vi "手动调试界面.vi"() -> ()   [LabVIEW 2016, in "质控单元.lvlib"]
uses:
  <vilib>/Utility/miscctls.llb/LVPointTypeDef.ctl
panel:
  in  "加标回收流程":bool
  in  "关闭":bool
  in  "总氮停止":bool
  in  "总氮排液":bool
  in  "总氮调试":bool
  in  "CODCr停止":bool
  in  "CODCr排液":bool
  in  "CODCr调试":bool
  in  "CODMn停止":bool
  in  "CODMn排液":bool
  in  "CODMn调试":bool
  in  "总磷停止":bool
  in  "总磷排液":bool
  in  "总磷调试":bool
  in  "氨氮停止":bool
  in  "氨氮排液":bool
  in  "氨氮调试":bool
  # "手动调试界面"
  # "氨氮模块"
  # "总磷模块"
  # "总氮模块"
  # "CODMn模块"
  # "CODCr模块"
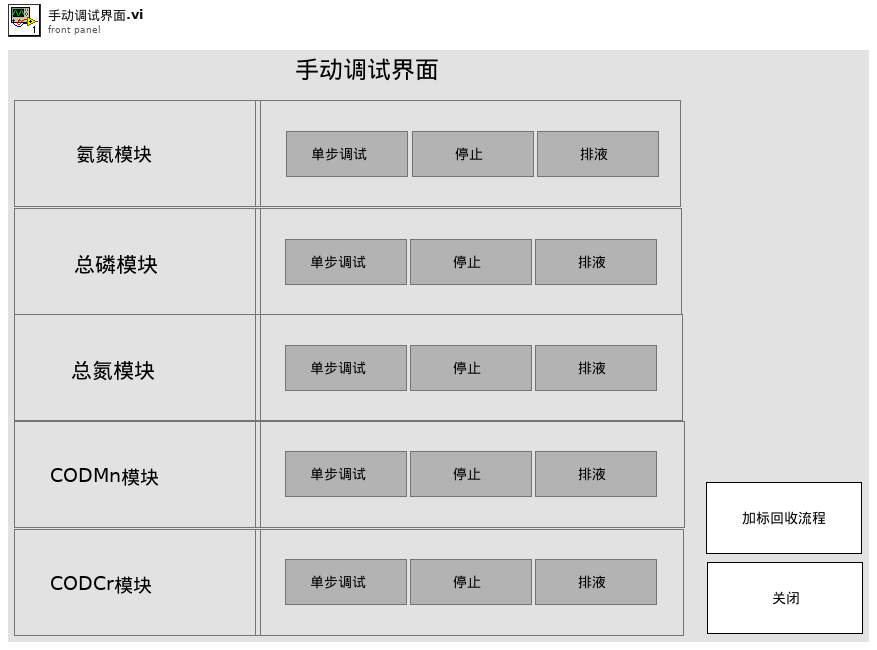
[diagram p1: front panel]
types:
  T1 = typedef "LVPointTypeDef.ctl" = cluster{"Horizontal":i16, "Vertical":i16}
  T2 = cluster{"氨氮":bool, "总磷":bool, "总氮":bool, "CODMn":bool, "CODCr":bool}
  T3 = enum32{"Bad", "Idle", "Run top level", "Running"}
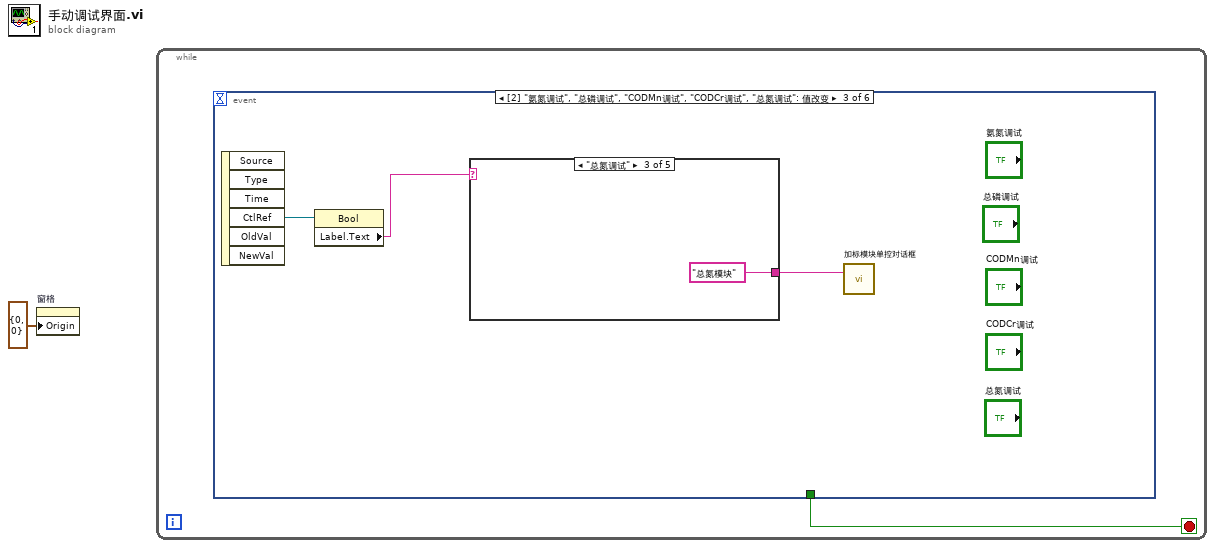
[diagram p0: block diagram]
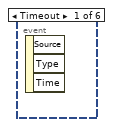
[diagram p2: hidden frame]
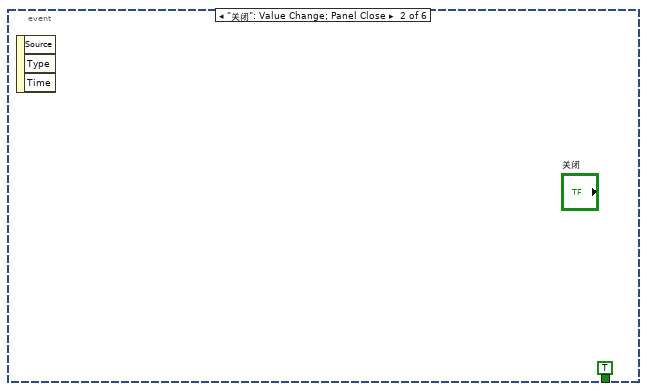
[diagram p3: hidden frame]
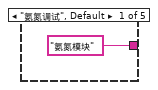
[diagram p4: hidden frame]
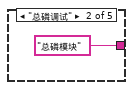
[diagram p5: hidden frame]
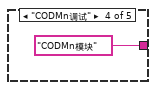
[diagram p6: hidden frame]
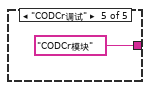
[diagram p7: hidden frame]
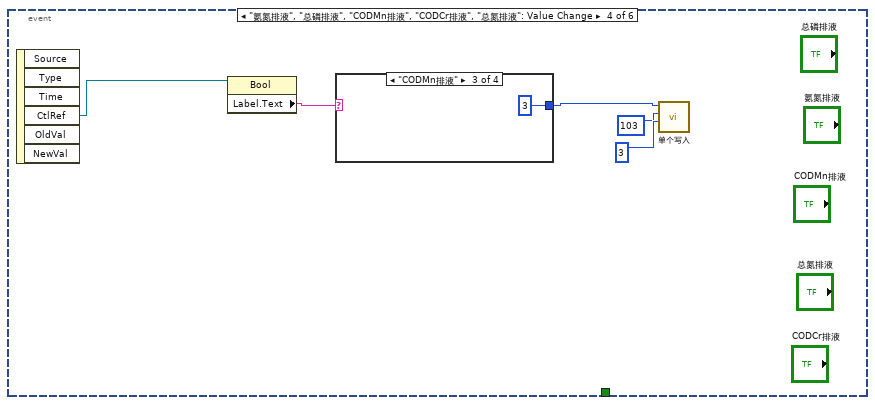
[diagram p8: hidden frame]
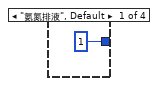
[diagram p9: hidden frame]
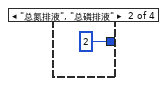
[diagram p10: hidden frame]
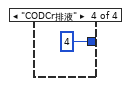
[diagram p11: hidden frame]
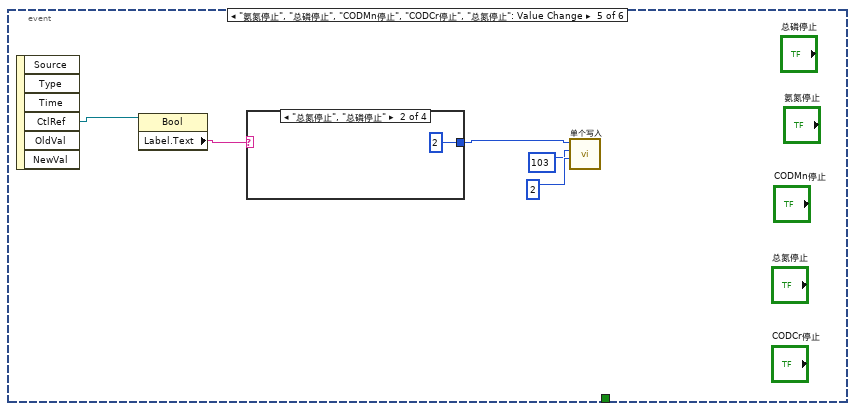
[diagram p12: hidden frame]
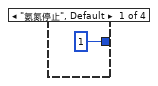
[diagram p13: hidden frame]
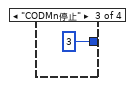
[diagram p14: hidden frame]
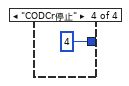
[diagram p15: hidden frame]
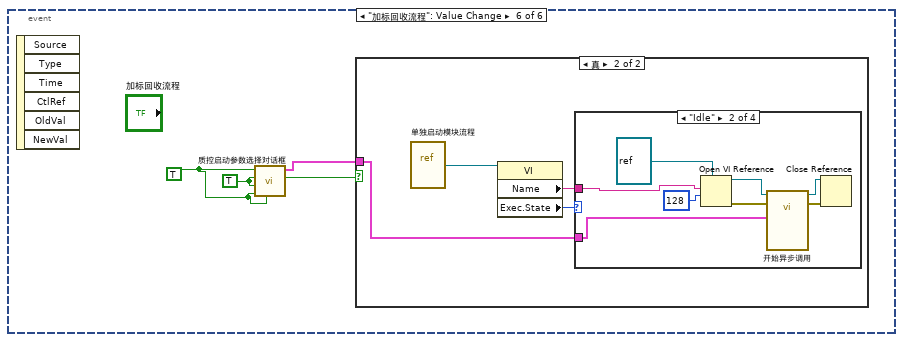
[diagram p16: hidden frame]
diagram:
  n1 = property on="窗格" class="Pane"("Origin"=T1 {"Horizontal"=0, "Vertical"=0} ("原点")) -> ()  [unwired: 2 in, 2 out]
  n2 = while {
    stop <- w2 stop-if-true
    n3 = event shown="[2] \"氨氮调试\", \"总磷调试\", \"CODMn调试\", \"CODCr调试\", \"总氮调试\": 值改变" {
      selector: _ -> [_ _ _ _ _ _]
      dyn-events: _ -> [_ _ _ _ _ _]
      timeout: _ -> [_ _ _ _ _ _]
      tunnel: [_ TRUE ("关闭") _ _ _ _] -> w2
      event Timeout {
        n4 = event-data() -> ()  [unwired: 1 in, 3 out]
      }
      event "关闭": Value Change; Panel Close {
        n5 = event-data() -> ()  [unwired: 1 in, 3 out]
      }
      event "氨氮调试", "总磷调试", "CODMn调试", "CODCr调试", "总氮调试": Value Change {
        n6 = event-data() -> ("CtlRef"=w5:refnum<vi>)  [unwired: 1 in, 5 out]
        n7 = property class="Bool"(reference=w5) -> ("Label.Text"=w4:string)  [unwired: 1 in, 2 out]
        n8 = case shown="\"总氮调试\"" w4 {
          tunnel: ["氨氮模块" ("标题") "总磷模块" ("标题") "总氮模块" ("标题") "CODMn模块" ("标题") "CODCr模块" ("标题")] -> w6
          frame "氨氮调试", Default {
          }
          frame "总磷调试" {
          }
          frame "总氮调试" {
          }
          frame "CODMn调试" {
          }
          frame "CODCr调试" {
          }
        }
        n9 = call "加标模块单控对话框.vi"("标题"=w6) -> ()  [unwired: 11 in]
      }
      event "氨氮排液", "总磷排液", "CODMn排液", "CODCr排液", "总氮排液": Value Change {
        n10 = event-data() -> ("CtlRef"=w12:refnum<vi>)  [unwired: 1 in, 5 out]
        n11 = property class="Bool"(reference=w12) -> ("Label.Text"=w16:string)  [unwired: 1 in, 2 out]
        n12 = case shown="\"CODMn排液\"" w16 {
          tunnel: [u8 1 ("Slave ID") u8 2 ("Slave ID") u8 3 ("Slave ID") u8 4 ("Slave ID")] -> w13
          frame "氨氮排液", Default {
          }
          frame "总氮排液", "总磷排液" {
          }
          frame "CODMn排液" {
          }
          frame "CODCr排液" {
          }
        }
        n13 = call "单个写入.vi"("value"=u16 3, "address"=u16 103, "Slave ID"=w13) -> ()  [unwired: 8 in, 1 out]
      }
      event "氨氮停止", "总磷停止", "CODMn停止", "CODCr停止", "总氮停止": Value Change {
        n14 = event-data() -> ("CtlRef"=w21:refnum<vi>)  [unwired: 1 in, 5 out]
        n15 = property class="Bool"(reference=w21) -> ("Label.Text"=w25:string)  [unwired: 1 in, 2 out]
        n16 = case shown="\"总氮停止\", \"总磷停止\"" w25 {
          tunnel: [u8 1 ("Slave ID") u8 2 ("Slave ID") u8 3 ("Slave ID") u8 4 ("Slave ID")] -> w22
          frame "氨氮停止", Default {
          }
          frame "总氮停止", "总磷停止" {
          }
          frame "CODMn停止" {
          }
          frame "CODCr停止" {
          }
        }
        n17 = call "单个写入.vi"("value"=u16 2, "address"=u16 103, "Slave ID"=w22) -> ()  [unwired: 8 in, 1 out]
      }
      event "加标回收流程": Value Change {
        w33 = TRUE ("总氮")
        w32 = TRUE ("氨氮")
        n18 = event-data() -> ()  [unwired: 1 in, 6 out]
        n19 = call "质控启动参数选择对话框.vi"("CODCr"=w32, "CODMn"=w32, "总氮"=w33, "总磷"=w33, "氨氮"=w32) -> ("确定启动"=w31:bool, "启动模块"=w30:T2)  [unwired: 4 in, 1 out]
        n20 = case shown="真" w31 {
          tunnel: w30 -> [_ w34]
          frame False {
          }
          frame True {
            n21 = vi-ref "单独启动模块流程.vi"() -> (w35:refnum<vi>)
            n22 = property class="VI"(reference=w35) -> ("Name"=w37:string, "Exec.State"=w36:T3)  [unwired: 1 in, 2 out]
            n23 = case shown="\"Idle\"" w36 {
              tunnel: w37 -> [_ w41 _ _]
              tunnel: w34 -> [_ w38 _ _]
              frame "Bad", Default {
              }
              frame "Idle" {
                n24 = Open VI Reference(type specifier VI Refnum (for type only)=refnum<vi> refnum ("类型说明符VI引用句柄（仅用于类型）"), vi path=w41, options=128 ("选项")) -> (vi reference=w45:refnum<vi>, error out=w40:errorcluster)  [unwired: 3 in]
                n25 = call-by-ref "开始异步调用"(reference=w45, error in=w40, "模块选择"=w38) -> (reference out=w44:refnum<vi>, error out=w39:errorcluster)  [unwired: 11 in]
                n26 = Close Reference(reference=w44, error in (no error)=w39) -> ()  [unwired: 1 out]
              }
              frame "Run top level" {
              }
              frame "Running" {
              }
            }
          }
        }
      }
    }
  }
